vi "07FootDAQLoop.vi"(7 "samples per channel":i32, 8 "error in (no error)":errorcluster, 11 "task in":refnum<k21>) -> (0 "error out":errorcluster, 3 "task out":refnum<k21>)   [LabVIEW 2020]
uses:
  07FootGlobals.vi
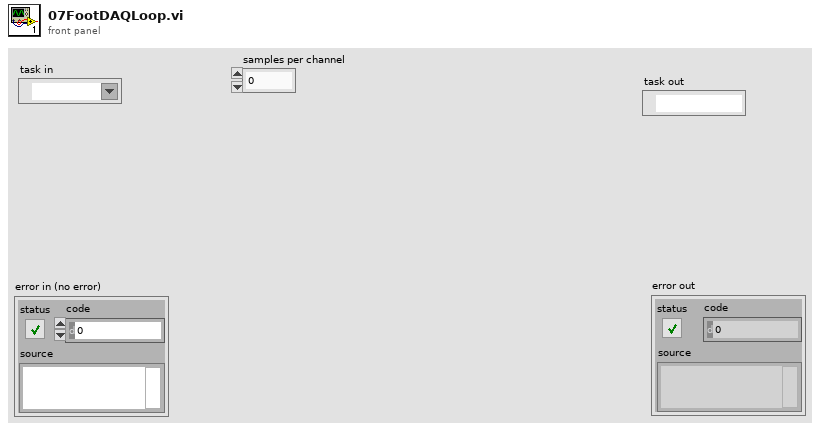
[diagram p1: front panel]
types:
  T1 = enum16{"Quit", "StartDAQ", "StopDAQ", "Starting", "Stopping"}
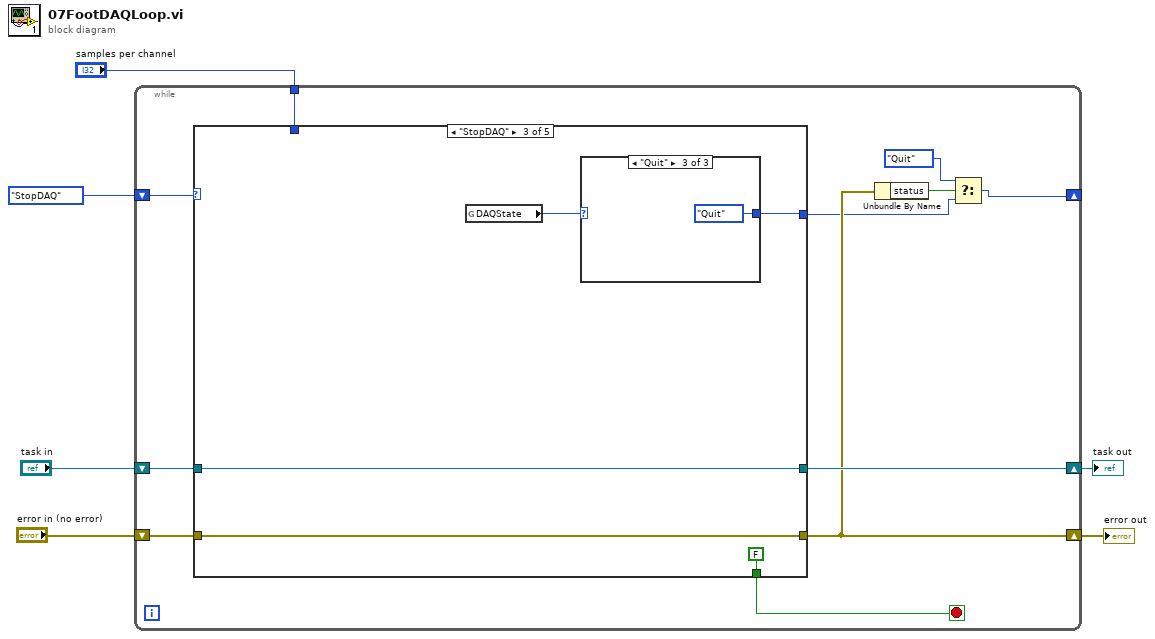
[diagram p0: block diagram]
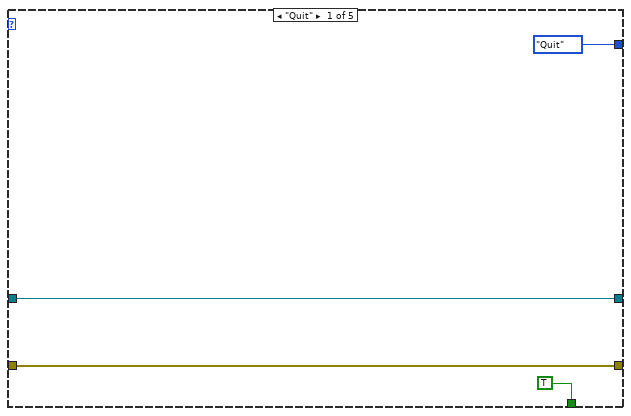
[diagram p2: hidden frame]
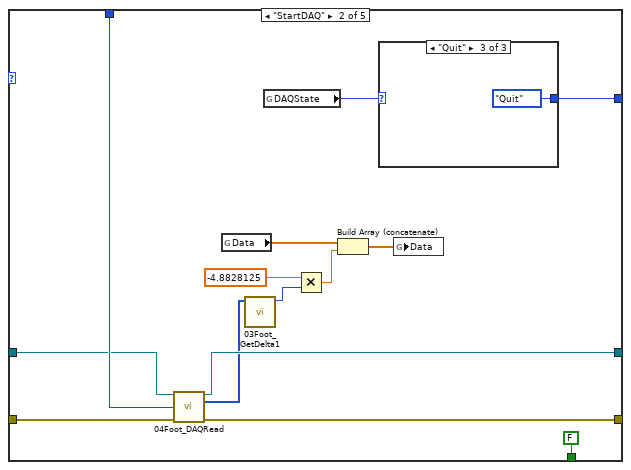
[diagram p3: hidden frame]
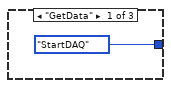
[diagram p4: hidden frame]
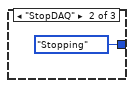
[diagram p5: hidden frame]
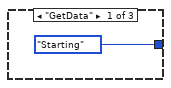
[diagram p6: hidden frame]
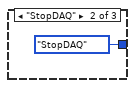
[diagram p7: hidden frame]
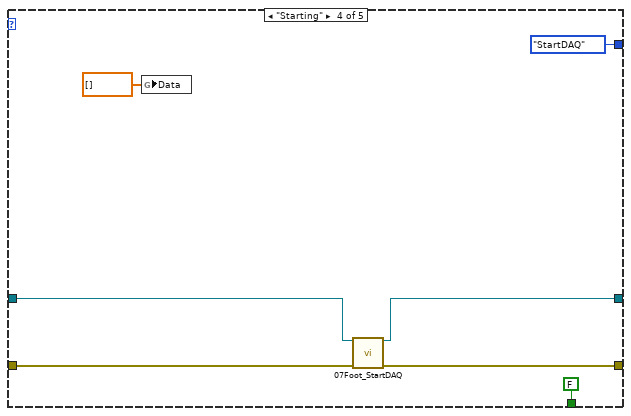
[diagram p8: hidden frame]
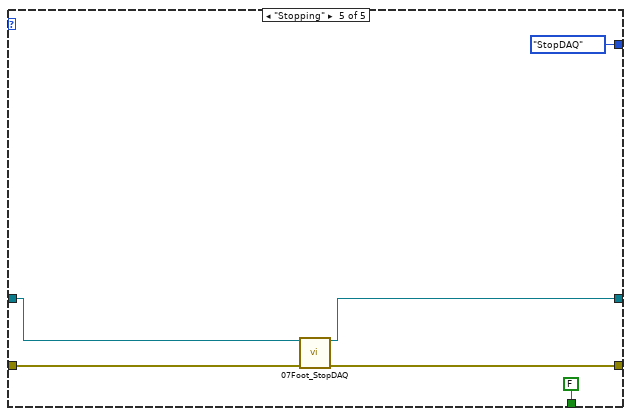
[diagram p9: hidden frame]
diagram:
  n1 = while {
    tunnel: "samples per channel" -> [w7]
    shift-right: [w8] -> _
    shift-left: T1."StopDAQ" -> [w17]
    shift-right: [w13] -> w2
    shift-left: "task in" -> [w15]
    shift-right: [w12] -> w1
    shift-left: "error in (no error)" -> [w16]
    stop <- w14 stop-if-true
    n2 = case shown="\"StopDAQ\"" w17 {
      tunnel: w16 -> [w20 w32 w41 w49 w56]
      tunnel: w15 -> [w21 w33 w42 w50 w57]
      tunnel: [TRUE FALSE FALSE FALSE FALSE] -> w14
      tunnel: [w21 w29 w42 w48 w55] -> w13
      tunnel: [w20 w28 w41 w47 w54] -> w12
      tunnel: [enum16{"Quit", "StartDAQ", "StopDAQ"}."Quit" w22 w39 T1."StartDAQ" T1."StopDAQ"] -> w9
      tunnel: w7 -> [_ w34 _ _ _]
      frame "Quit" {
      }
      frame "StartDAQ" {
        n3 = call "04Foot_DAQRead.vi"("task/channels in"=w33, "number of samples per channel"=w34, "error in"=w32) -> ("task out"=w29:refnum<k21>, "data"=w27:u8[], "error out"=w28:errorcluster)  [unwired: 10 in]
        n4 = global read "07FootGlobals.vi" "Data"() -> (w26:dbl[])
        n5 = call "03Foot_GetDelta1.vi"("Array"=w27) -> ("Wave1 Data"=w30:i32)  [unwired: 10 in]
        n6 = global read "07FootGlobals.vi" "DAQState"() -> (w23:enum16{"GetData", "StopDAQ", "Quit"})
        n7 = Multiply(x=-4.8828125, y=w30) -> (x*y=w25:dbl)
        n8 = Build Array (concatenate)(w26, w25) -> (w24:dbl[])
        n9 = case shown="\"Quit\"" w23 {
          tunnel: [T1."StartDAQ" T1."Stopping" T1."Quit"] -> w22
          frame "GetData" {
          }
          frame "StopDAQ" {
          }
          frame "Quit" {
          }
        }
        n10 = global write "07FootGlobals.vi" "Data"(w24) -> ()
      }
      frame "StopDAQ" {
        n11 = global read "07FootGlobals.vi" "DAQState"() -> (w40:enum16{"GetData", "StopDAQ", "Quit"})
        n12 = case shown="\"Quit\"" w40 {
          tunnel: [T1."Starting" T1."StopDAQ" T1."Quit"] -> w39
          frame "GetData" {
          }
          frame "StopDAQ" {
          }
          frame "Quit" {
          }
        }
      }
      frame "Starting" {
        n13 = global write "07FootGlobals.vi" "Data"(dbl[] [] ("Data")) -> ()
        n14 = call "07Foot_StartDAQ.vi"("task/channels in"=w50, "error in"=w49) -> ("task out"=w48:refnum<k21>, "error out"=w47:errorcluster)  [unwired: 12 in]
      }
      frame "Stopping" {
        n15 = call "07Foot_StopDAQ.vi"("task/channels in"=w57, "error in"=w56) -> ("task out"=w55:refnum<k21>, "error out"=w54:errorcluster)  [unwired: 12 in]
      }
    }
    n16 = Unbundle By Name(w12) -> ("status"=w11:bool)
    n17 = Select(t=enum16{"Quit", "StartDAQ", "StopDAQ"}."Quit", s=w11, f=w9) -> (s? t:f=w8:T1)
  }
  "error out" <- w1
  "task out" <- w2
